vi "Get FPGA Sync Flag.vi"(8 "error in (no error)":errorcluster, 10 "FPGA Name":string, 11 "Tamer in":refnum<class "Tamer.lvclass">) -> (0 "error out":errorcluster, 2 "FPGA Sync Flag":bool, 3 "Tamer out":refnum<class "Tamer.lvclass">)   [LabVIEW 2020, in "Tamer.lvlib" / "Tamer.lvclass"]
uses:
  Tamer.lvclass
  Tamer.lvclass/Tamer.ctl
  Ancestor/Ancestor/Ancestor.lvclass/Ancestor.ctl
  FGV/Error Memory/Get Error Description.vi
  Support VIs/Get PC name.vi
  Ancestor/Ancestor/Read ID.vi
  Support VIs/Get Class Name.vi
  <vilib>/Utility/error.llb/Clear Errors.vi
  FGV/Error Memory/Error Memory Core.vi
  <vilib>/AdvancedString/Delimited String to 1D String Array.vi
  Support VIs/Circus Root Path.vi
  FGV/Error Memory/Error Crt Lvl checker.vi
  FGV/Error Memory/Error Memory Core.vi/40c8088d-b597-4017-91af-faa98e00292e.vi
  FGV/Error Memory/Error Memory Core.vi/d4a3ab98-063c-4e44-b43d-fbdcfe6c2be2.vi
  Support VIs/Global Memory.vi
  <vilib>/Utility/LVClass/Get LV Class Name.vi
  Support VIs/Is in Packed Library.vi
  Support VIs/TALOS Root path.vi
  Support VIs/Read CSV worksheet.vi
  Support VIs/Global Constants.vi
  <vilib>/Utility/error.llb/General Error Handler.vi
  Ancestor/Ancestor/Ancestor.lvclass
  <vilib>/Comparison/Equal/Equal Functor/Equal Functor.lvclass
  TALOS.lvlib
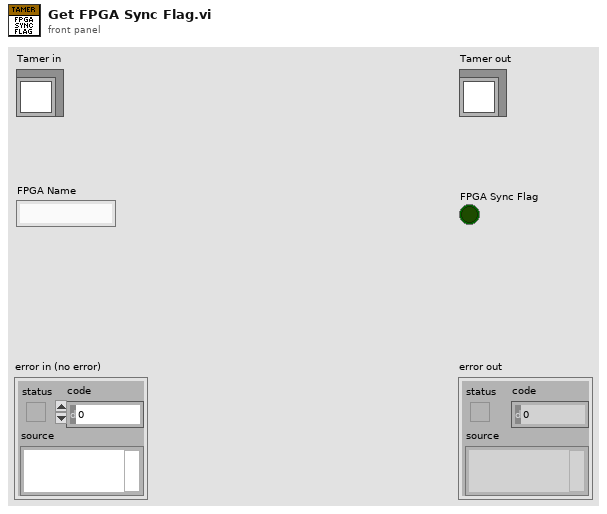
[diagram p1: front panel]
types:
  T1 = typedef "TALOS.lvlib/Run Utilities.lvlib/Synchronize FPGA Cluster.ctl" = cluster{"Status":bool, "FPGA Name":string}
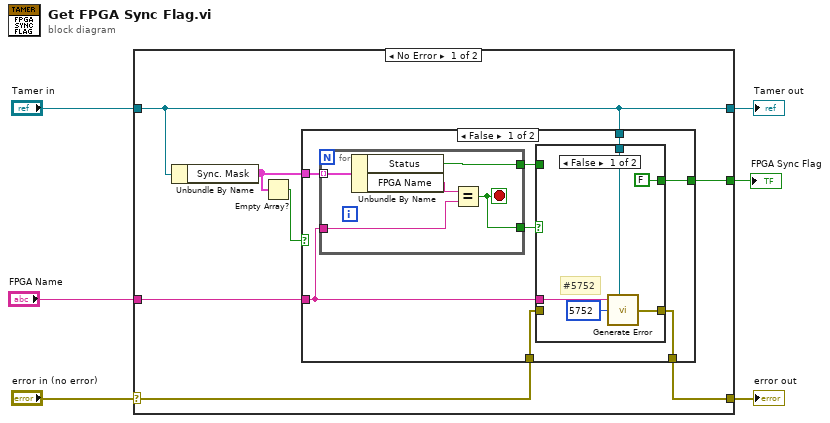
[diagram p0: block diagram]
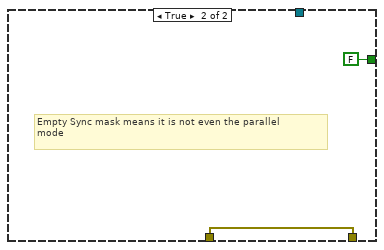
[diagram p3: hidden frame]
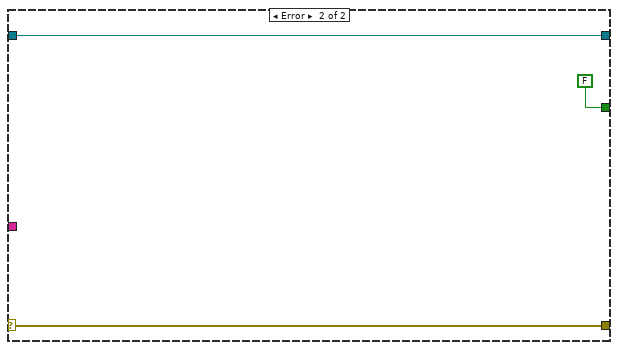
[diagram p4: hidden frame]
diagram:
  n1 = case shown="No Error" "error in (no error)" {
    selector: "error in (no error)" -> [w9 w38]
    tunnel: [w11 w38] -> w5
    tunnel: [w12 w37] -> w3
    tunnel: "Tamer in" -> [w12 w37]
    tunnel: "FPGA Name" -> [w10 _]
    tunnel: [w13 FALSE ("f")] -> w1
    frame No Error {
      n2 = Unbundle By Name(w12) -> ("Sync. Mask"=w8:T1[])
      n3 = Empty Array?(array=w8) -> (empty?=w7:bool)
      n4 = case shown="False" w7 {
        tunnel: [w19 FALSE ("Status")] -> w13
        tunnel: w12 -> [w18 _]
        tunnel: [w17 w34] -> w11
        tunnel: w10 -> [w14 _]
        tunnel: w9 -> [w16 w34]
        tunnel: w8 -> [w15 _]
        frame False {
          n5 = for {
            tunnel: w15 -> [w26] mode=indexing
            tunnel: w14 -> [w24]
            tunnel: [w22] -> w20
            tunnel: [w23] -> w21
            stop <- w23 stop-if-true
            n6 = Unbundle By Name(w26) -> ("Status"=w22:bool, "FPGA Name"=w25:string)
            n7 = Equal?(x=w25, y=w24) -> (x = y?=w23:bool)
          }
          n8 = case shown="False" w21 {
            tunnel: w20 -> [_ w33]
            tunnel: [FALSE w33] -> w19
            tunnel: w18 -> [w30 _]
            tunnel: [w29 w32] -> w17
            tunnel: w14 -> [w27 _]
            tunnel: w16 -> [_ w32]
            frame False {
              # "#5752"
              n9 = call "Generate Error.vi"("Optional String"=w27, "Class"=w30, "Error Code"=5752) -> ("error out"=w29:errorcluster)  [unwired: 4 in]
            }
            frame True {
            }
          }
        }
        frame True {
          # "Empty Sync mask means it is not even the parallel\nmode"
        }
      }
    }
    frame Error {
    }
  }
  "error out" <- w5
  "Tamer out" <- w3
  "FPGA Sync Flag" <- w1
